vi "name.get.vi"(11 "test-group in":refnum<class "test-group.lvclass">) -> (2 "name":string, 3 "test-group out":refnum<class "test-group.lvclass">)   [LabVIEW 2020, in "test-group.lvclass"]
uses:
  test-group.lvclass
  test-group.lvclass/test-group.ctl
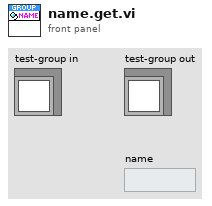
[diagram p1: front panel]
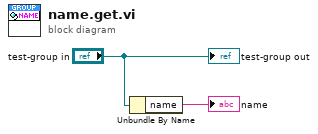
[diagram p0: block diagram]
diagram:
  n1 = Unbundle By Name("test-group in") -> ("name"=→"name":string)
  "test-group out" <- "test-group in"
